vi "Assign GPIO.vi"(8 "error in (no error)":errorcluster, 9 "SDA":T1=-1, 10 "SCL":T1=-1, 11 "I2C in":refnum<class "I2C.lvclass">) -> (0 "error out":errorcluster, 3 "I2C out":refnum<class "I2C.lvclass">)   [LabVIEW 2024, in "CTI.lvlib" / "I2C.lvclass"]
uses:
  I2C.lvclass
  GPIO Number.ctl
  I2C.lvclass/I2C.ctl
  CTI.lvlib
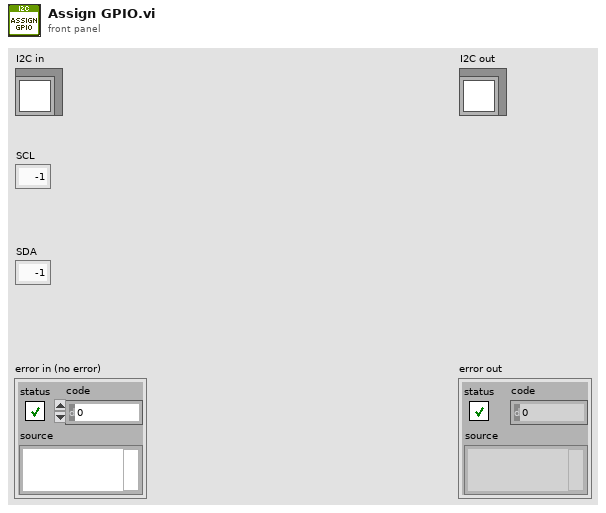
[diagram p1: front panel]
types:
  T1 = typedef "CTI.lvlib/GPIO Number.ctl" = i8
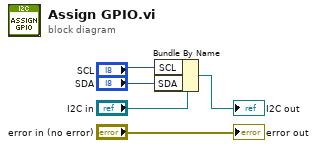
[diagram p0: block diagram]
diagram:
  n1 = Bundle By Name(cluster="I2C in", "SCL"="SCL", "SDA"="SDA") -> (→"I2C out":refnum<class "I2C.lvclass">)
  "error out" <- "error in (no error)"
